vi "even_noteven.vi"() -> ()   [LabVIEW 2013]
panel:
  out "valeur sélectionnée":string
  out "Not even":bool
  out "Even":bool
  out "Not Even":bool
  out "Even":bool
  in  "Numérique":dbl
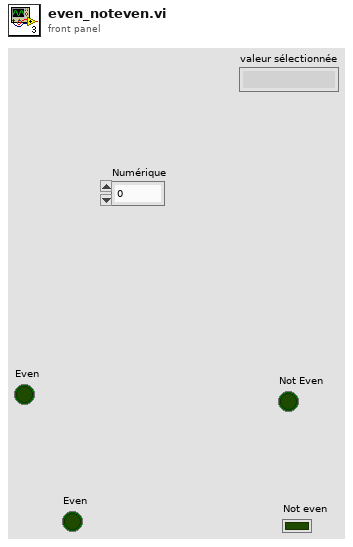
[diagram p1: front panel]
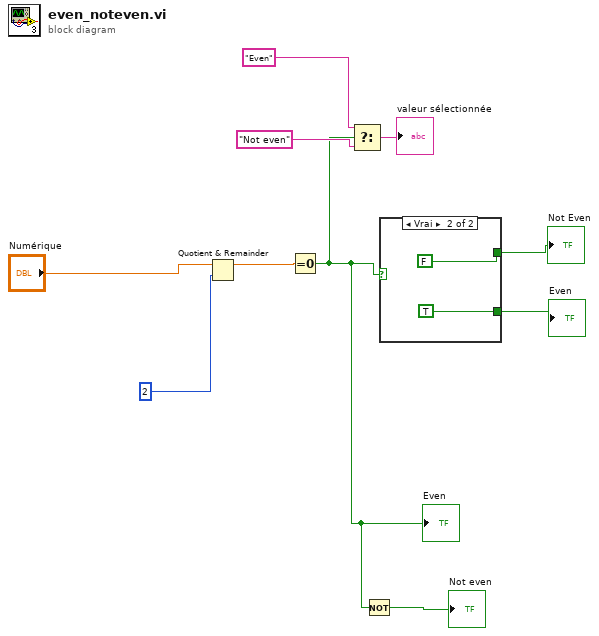
[diagram p0: block diagram]
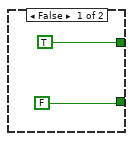
[diagram p2: hidden frame]
diagram:
  n1 = Quotient & Remainder(x="Numérique", y=2) -> (x-y*floor(x/y)=w8:dbl)  [unwired: 1 out]
  n2 = Equal To 0?(x=w8) -> (x = 0?=w2:bool)
  "Even" <- w2
  n3 = Select(t="Even", s=w2, f="Not even") -> (s? t:f=→"valeur sélectionnée":string)
  n4 = Not(x=w2) -> (.not. x?=→"Not even":bool)
  n5 = case shown="Vrai" w2 {
    tunnel: [FALSE TRUE] -> w7
    tunnel: [TRUE FALSE] -> w6
    frame False {
    }
    frame True {
    }
  }
  "Even" <- w7
  "Not Even" <- w6
